vi "Terminal-PressureSystemLubricateUnit-SwitchSetter.vi"(8 "error in (no error)":errorcluster caption="错误输入（无错误）", 10 "启停":bool=TRUE, 11 "operation timeout (ms)":i32=5000 caption="操作超时（5000毫秒）") -> (0 "error out":errorcluster caption="错误输出")   [LabVIEW 2014]
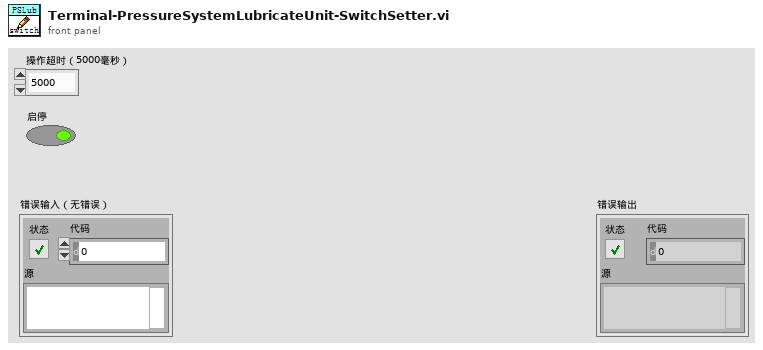
[diagram p1: front panel]
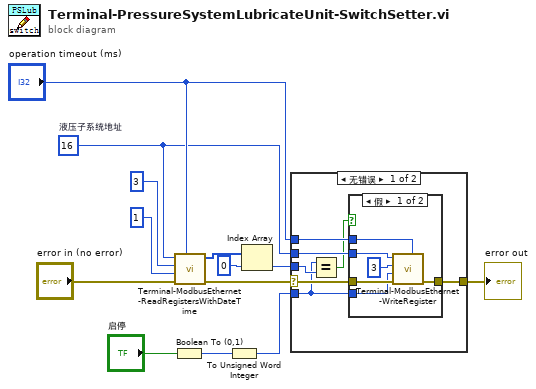
[diagram p0: block diagram]
diagram:
  w7 = u8 16  # 液压子系统地址
  n1 = Boolean To (0,1)(Boolean="启停") -> (0, 1=w12:i16)
  n2 = call "Terminal-ModbusEthernet-ReadRegistersWithDateTime.vi"("read operation timeout (ms)"="operation timeout (ms)", "error in"="error in (no error)", "number of holding registers"=u16 1 ("address"), "starting address"=u16 3, "unit ID"=w7) -> ("error out"=w10:errorcluster, "register values"=w3:u16[])  [unwired: 4 in, 1 out]
  n3 = To Unsigned Word Integer(number=w12) -> (unsigned 16bit integer=w11:u16)
  n4 = Index Array(array=w3, index=0 ("索引")) -> (element=w1:u16)
  n5 = case shown="无错误" w10 {
    selector: w10 -> [w18 w28]
    tunnel: "operation timeout (ms)" -> [w20 _]
    tunnel: [w19 w28] -> w13
    tunnel: w7 -> [w17 _]
    tunnel: w11 -> [w15 _]
    tunnel: w1 -> [w16 _]
    frame No Error {
      n6 = Equal?(x=w15, y=w16) -> (x = y?=w14:bool)
      n7 = case shown="假" w14 {
        tunnel: w20 -> [w26 _]
        tunnel: [w25 w27] -> w19
        tunnel: w18 -> [w24 w27]
        tunnel: w17 -> [w23 _]
        tunnel: w15 -> [w22 _]
        frame False {
          n8 = call "Terminal-ModbusEthernet-WriteRegister.vi"("write operation timeout (ms)"=w26, "error in"=w24, "holding register value"=w22, "address"=u16 3, "unit ID"=w23) -> ("error out"=w25:errorcluster)  [unwired: 6 in]
        }
        frame True {
        }
      }
    }
    frame Error {
    }
  }
  "error out" <- w13
